vi "Set LabVIEW Array Parameter by Expression.vi"(0 "Measurement Interface in":refnum<class "Measurement Interface.lvclass">, 5 "Step In":refnum<k7>, 7 "LabVIEW Parameter to Set":string, 9 "Array of Expresssions":string[](array[string]), 11 "error in (no error)":errorcluster) -> (4 "Measurement Interface out":refnum<class "Measurement Interface.lvclass">, 6 "Step Out":refnum<k7>, 15 "error out":errorcluster)   [LabVIEW 2016, in "Measurement Interface.lvlib" / "Measurement Interface.lvclass"]
uses:
  Measurement Interface.lvclass
  Measurement Interface.lvclass/Measurement Interface.ctl
  Engine Reference/Read Engine Reference.vi
  Plugins/TestStand API Tools (TSAT).lvlibp/Step Actions/TSAT Step Actions.lvlib
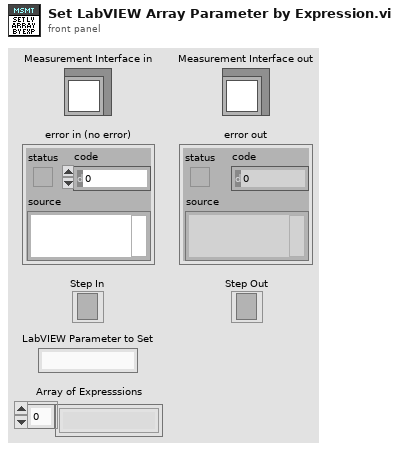
[diagram p1: front panel]
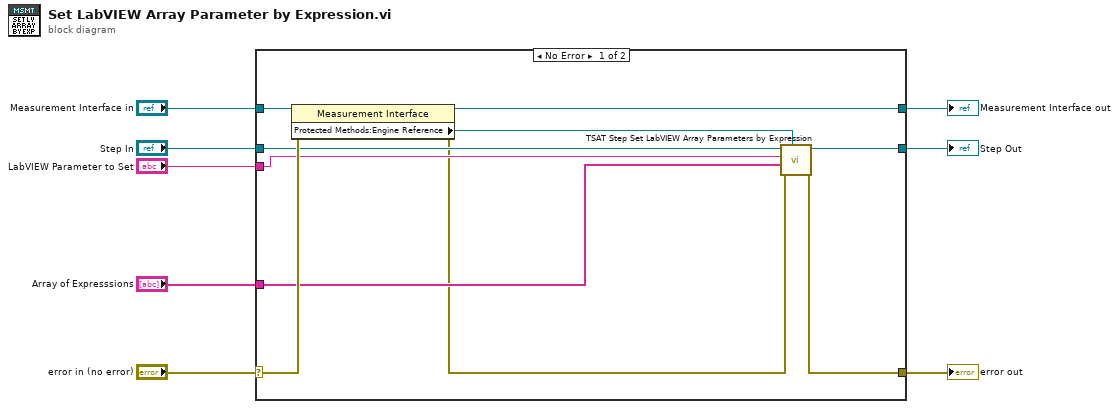
[diagram p0: block diagram]
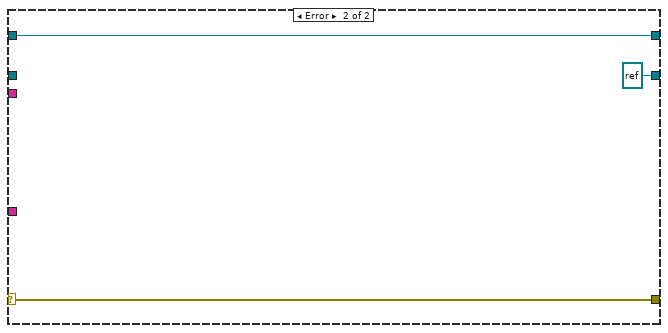
[diagram p2: hidden frame]
diagram:
  n1 = case shown="No Error" "error in (no error)" {
    selector: "error in (no error)" -> [w18 w21]
    tunnel: [w17 w21] -> w1
    tunnel: [w10 w20] -> w3
    tunnel: "Measurement Interface in" -> [w11 w20]
    tunnel: "Array of Expresssions" -> [w16 _]
    tunnel: "LabVIEW Parameter to Set" -> [w13 _]
    tunnel: "Step In" -> [w15 _]
    tunnel: [w14 refnum<k7> refnum ("Step Out")] -> w6
    frame No Error {
      n2 = property class="Measurement Interface"(reference=w11, error in=w18) -> (reference out=w10:refnum<class "Measurement Interface.lvclass">, error out=w12:errorcluster, "Protected Methods:Engine Reference"=w9:refnum<k7>)
      n3 = call "TSAT Step Set LabVIEW Array Parameters by Expression.vi"("Engine In"=w9, "Error In"=w12, "Value Expressions"=w16, "Parameter to Set"=w13, "Step In"=w15) -> ("Error Out"=w17:errorcluster, "Step Out"=w14:refnum<k7>)  [unwired: 5 in]
    }
    frame Error {
    }
  }
  "error out" <- w1
  "Measurement Interface out" <- w3
  "Step Out" <- w6
